vi "test-quintic-spline-02.vi"() -> (3 "Test Passed":bool)   [LabVIEW 2019]
uses:
  <vilib>/Rock Robotics/WPI/ThirdParty/JAS_Junk/TrajLib/POSEwCURVATURE.ctl
  <vilib>/Rock Robotics/WPI/ThirdParty/JAS_Junk/TrajLib/POSE2D.ctl
  <vilib>/Rock Robotics/WPI/ThirdParty/JAS_Junk/TrajLib/TRANSLATION2D.ctl
  <vilib>/Rock Robotics/WPI/ThirdParty/JAS_Junk/TrajLib/ROTATION2D.ctl
  <vilib>/Rock Robotics/WPI/ThirdParty/JAS_Junk/TrajLib/Rotation2d_CreateAngle.vi
  <vilib>/Rock Robotics/WPI/ThirdParty/JAS_Junk/TrajLib/Translation2d_Create.vi
  <vilib>/Rock Robotics/WPI/ThirdParty/JAS_Junk/TrajLib/Util_CalcDist.vi
  <vilib>/Rock Robotics/WPI/ThirdParty/JAS_Junk/TrajLib/Trajectory_Library.lvlib
panel:
  out "XY Graph":cluster{dbl[], dbl[]}(graph)
  out "Numb\nWaypoints":i32
  out "All Interior \nwayPoints\nFound (True)":bool
  out "end rot = 0":dbl
  out "end y = 0":dbl
  out "end x = 0":dbl
  out "start rot = 0":dbl
  out "start y = 0":dbl
  out "start x = 0":dbl
  out "max dtheta < 0.0872":dbl
  out "max dy < 0.00127":dbl
  out "max dx  < 0.127":dbl
  out "Overall Error":errorcluster
  out "Elements":i32
  out "Create Spline Error":errorcluster
  out "SplinePoses\nWCurve":T1[](array[typedef]) {"POSE"."ROTATION"."SIN" format="%13.4f"; "POSE"."ROTATION"."COS" format="%13.4f"; "POSE"."ROTATION"."VALUE" format="%13.4f"; "POSE"."TRANSLATION"."Y" format="%14.3f"; "POSE"."TRANSLATION"."X" format="%14.3f"}
  out "Elapsed Time":dbl
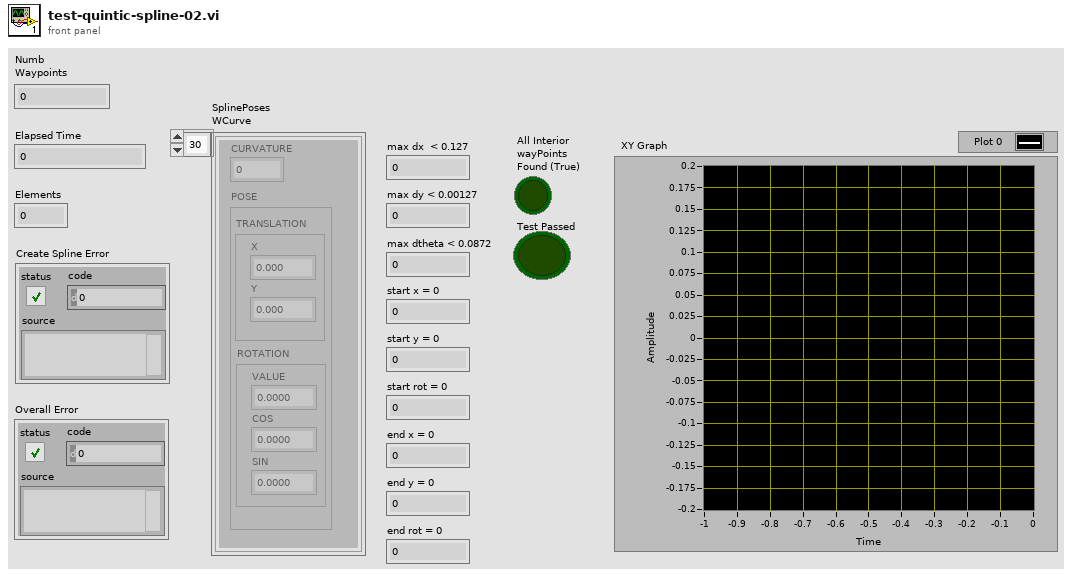
[diagram p1: front panel]
types:
  T1 = typedef "Trajectory_Library.lvlib/POSEwCURVATURE.ctl" = cluster{"CURVATURE":dbl, "POSE":T2}
  T2 = typedef "Trajectory_Library.lvlib/POSE2D.ctl" = cluster{"TRANSLATION":T3, "ROTATION":T4}
  T3 = typedef "Trajectory_Library.lvlib/TRANSLATION2D.ctl" = cluster{"X":dbl, "Y":dbl}
  T4 = typedef "Trajectory_Library.lvlib/ROTATION2D.ctl" = cluster{"VALUE":dbl, "COS":dbl, "SIN":dbl}
  T5 = typedef "Trajectory_Library.lvlib/SPLINE.ctl" = cluster{"Degree":i32, "Coefficients":T6}
  T6 = typedef "NI_Matrix.lvlib/RealMatrix.ctl" = dbl[][]
  T7 = typedef "Trajectory_Library.lvlib/TWIST2D.ctl" = cluster{"dX":dbl, "dY":dbl, "dTHETA":dbl}
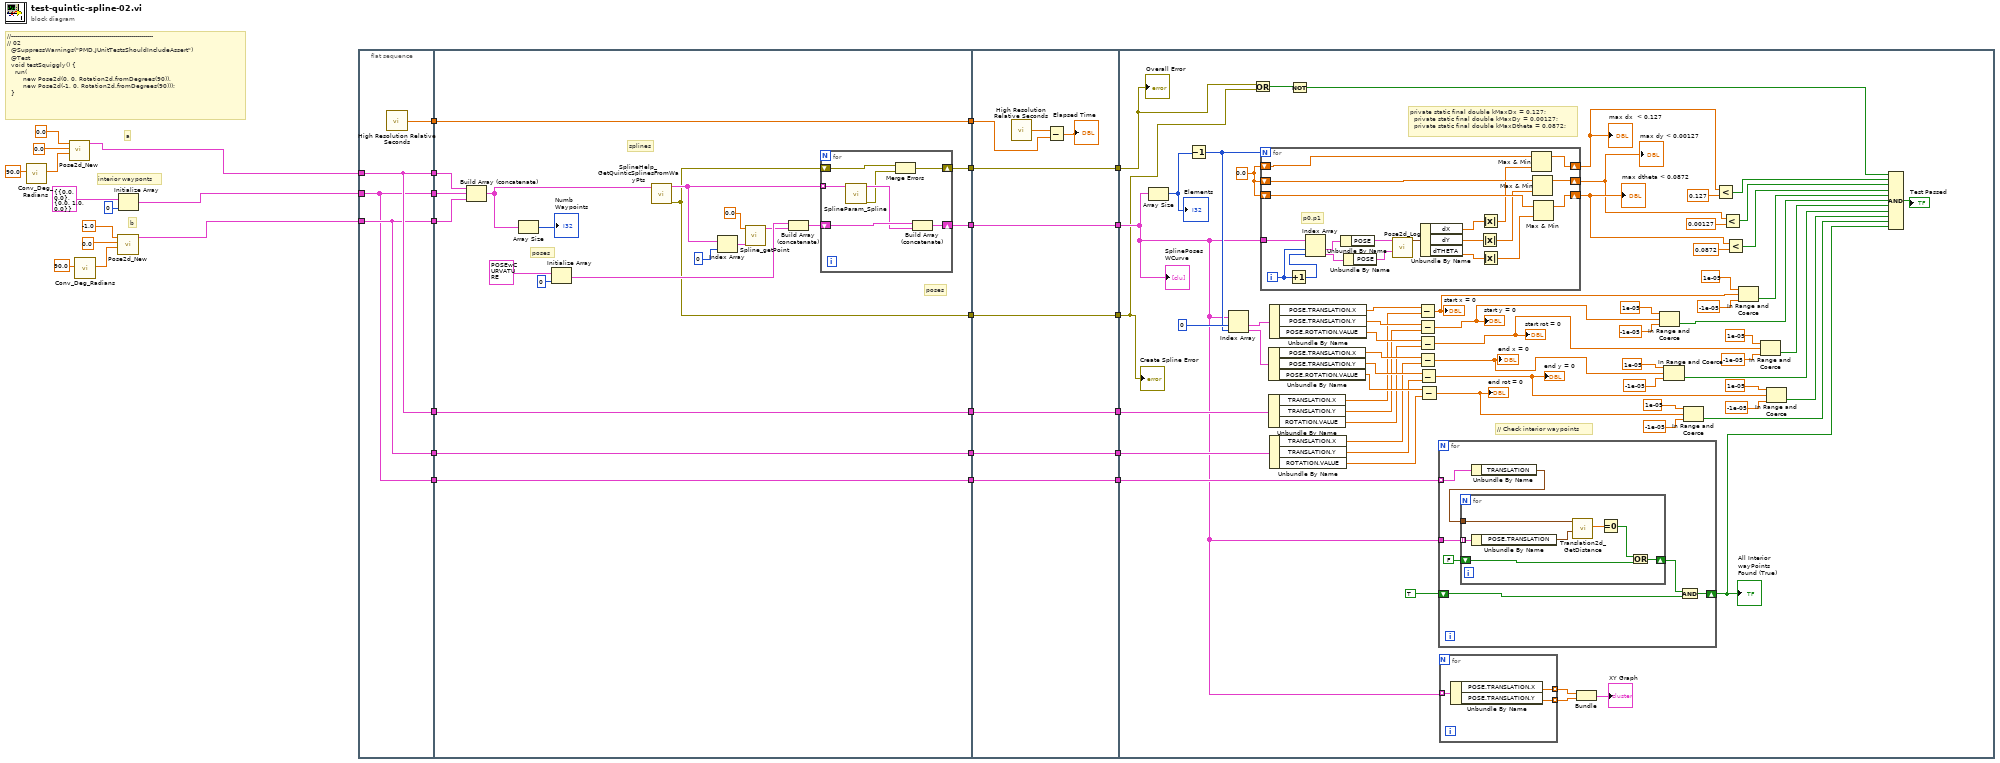
[diagram p0: block diagram]
diagram:
  # "interior wayponts"
  # "b"
  # "a"
  # "//-----------------------------------------------------------------------\n// 02\n  @SuppressWarnings(\"PMD.JUnitTestsShouldIncludeAssert\")\n  @Test\n  void testSquiggly() {\n    run(\n        new Pose2d(0, 0, Rotation2d.fromDegrees(90)),\n        new Pose2d(-1, 0, Rotation2d.fromDegrees(90)));\n  }"
  n1 = call <vilib>:"Conv_Deg_Radians.vi"("Degress"=90.0) -> ("Radians"=w6:dbl)  [unwired: 10 in]
  n2 = call <vilib>:"Pose2d_New.vi"("Heading"=w6, "Y"=0.0, "X"=0.0) -> ("out POSe"=w3:T2)  [unwired: 8 in]
  n3 = call <vilib>:"Conv_Deg_Radians.vi"("Degress"=90.0) -> ("Radians"=w9:dbl)  [unwired: 10 in]
  n4 = call <vilib>:"Pose2d_New.vi"("Heading"=w9, "Y"=0.0, "X"=-1.0) -> ("out POSe"=w1:T2)  [unwired: 8 in]
  n5 = Initialize Array(T2 {"TRANSLATION"={"X"=0.0, "Y"=0.0}, "ROTATION"={"VALUE"=0.0, "COS"=1.0, "SIN"=0.0}} ("POSE"), 0 ("dimension size")) -> (w2:T2[])
  n6 = flat-sequence {
    tunnel: w3 -> [w36]
    tunnel: [w36] -> w33
    tunnel: w1 -> [w35]
    tunnel: [w35] -> w32
    tunnel: [w37] -> w31
    tunnel: [w36] -> w23
    tunnel: [w35] -> w20
    tunnel: [w34] -> w15
    tunnel: w2 -> [w34]
    tunnel: [w34] -> w14
    tunnel: w33 -> [w42]
    tunnel: w32 -> [w41]
    tunnel: [w58] -> w30
    tunnel: w31 -> [w58]
    tunnel: [w48] -> w29
    tunnel: [w47] -> w27
    tunnel: [w46] -> w25
    tunnel: w23 -> [w45]
    tunnel: [w45] -> w22
    tunnel: w20 -> [w44]
    tunnel: [w44] -> w19
    tunnel: [w43] -> w16
    tunnel: w15 -> [w43]
    tunnel: w14 -> [w39]
    tunnel: w30 -> [w74]
    tunnel: w29 -> [w73]
    tunnel: [w73] -> w28
    tunnel: w27 -> [w72]
    tunnel: [w72] -> w26
    tunnel: w25 -> [w71]
    tunnel: [w71] -> w24
    tunnel: w22 -> [w68]
    tunnel: [w68] -> w21
    tunnel: w19 -> [w67]
    tunnel: [w67] -> w18
    tunnel: [w66] -> w17
    tunnel: w16 -> [w66]
    tunnel: w28 -> [w115]
    tunnel: w26 -> [w102]
    tunnel: w24 -> [w101]
    tunnel: w21 -> [w137]
    tunnel: w18 -> [w136]
    tunnel: w17 -> [w119]
    frame #0 {
      n7 = call <vilib>:"High Resolution Relative Seconds.vi"() -> ("relative seconds"=w37:dbl)
    }
    frame #1 {
      # "poses"
      # "poses"
      # "splines"
      n8 = Build Array (concatenate)(w42, w39, w41) -> (w38:T2[])
      n9 = Array Size(array=w38) -> (size(s)=→"Numb\nWaypoints":i32)
      n10 = Initialize Array(T1 {"CURVATURE"=0.0, "POSE"={"TRANSLATION"={"X"=0.0, "Y"=0.0}, "ROTATION"={"VALUE"=0.0, "COS"=1.0, "SIN"=0.0}}} ("POSEwCURVATURE"), 0 ("dimension size")) -> (w52:T1[])
      n11 = call <vilib>:"SplineHelp_GetQuinticSplinesFromWayPts.vi"("WayPoints"=w38) -> ("out Error"=w47:errorcluster, "Splines"=w49:T5[])  [unwired: 9 in]
      n12 = Index Array(array=w49, index=0) -> (element=w54:T5)
      n13 = call <vilib>:"Spline_getPoint.vi"("inputSPLINE"=w54, "Time"=0.0) -> ("POSEwCURVATURE"=w51:T1)  [unwired: 9 in]
      n14 = Build Array (concatenate)(w52, w51) -> (w50:T1[])
      n15 = for {
        shift-right: [w62] -> w48
        shift-left: w50 -> [w64]
        tunnel: w49 -> [w65] mode=indexing
        shift-right: [w60] -> w46
        shift-left: w47 -> [w61]
        n16 = call <vilib>:"SplineParam_Spline.vi"("inputSPLINE"=w65) -> ("error out"=w59:errorcluster, "outputPOSEwCURVATURE"=w63:T1[])  [unwired: 9 in]
        n17 = Merge Errors(w61, w59) -> (w60:errorcluster)
        n18 = Build Array (concatenate)(w64, w63) -> (w62:T1[])
      }
    }
    frame #2 {
      n19 = call <vilib>:"High Resolution Relative Seconds.vi"() -> ("relative seconds"=w69:dbl)
      n20 = Subtract(x=w69, y=w74) -> (x-y=→"Elapsed Time":dbl)
    }
    frame #3 {
      w138 = 0.0
      # "// Check interior waypoints"
      # "private static final double kMaxDx = 0.127;\n  private static final double kMaxDy = 0.00127;\n  private static final double kMaxDtheta = 0.0872;"
      n21 = Array Size(array=w115) -> (size(s)=w139:i32)
      "Elements" <- w139
      n22 = Decrement(x=w139) -> (x-1=w134:i32)
      n23 = Index Array(array=w115, index #1=0 ("index"), index #2=w134) -> (element #1=w133:T1, element #2=w132:T1)
      n24 = Or(x=w101, y=w102) -> (x .or. y?=w103:bool)
      n25 = for {
        N: w134 -> [_]
        tunnel: w115 -> [w174]
        shift-right: [w165] -> w107
        shift-left: w138 -> [w162]
        shift-right: [w163] -> w109
        shift-left: w138 -> [w160]
        shift-right: [w164] -> w108
        shift-left: w138 -> [w161]
        i -> [w176]
        # "p0,p1"
        n26 = Increment(x=w176) -> (x+1=w175:i32)
        n27 = Index Array(array=w174, index #1=w176, index #2=w175) -> (element #1=w173:T1, element #2=w172:T1)
        n28 = Unbundle By Name(w173) -> ("POSE"=w171:T2)
        n29 = Unbundle By Name(w172) -> ("POSE"=w170:T2)
        n30 = call <vilib>:"Pose2d_Log.vi"("end POSE"=w170, "in POSE"=w171) -> ("out TWIST"=w169:T7)  [unwired: 9 in]
        n31 = Unbundle By Name(w169) -> ("dX"=w166:dbl, "dY"=w167:dbl, "dTHETA"=w168:dbl)
        n32 = Absolute Value(x=w167) -> (abs(x)=w158:dbl)
        n33 = Absolute Value(x=w166) -> (abs(x)=w159:dbl)
        n34 = Absolute Value(x=w168) -> (abs(x)=w157:dbl)
        n35 = Max & Min(x=w162, y=w159) -> (max(x,y)=w165:dbl)  [unwired: 1 out]
        n36 = Max & Min(x=w161, y=w158) -> (max(x,y)=w164:dbl)  [unwired: 1 out]
        n37 = Max & Min(x=w160, y=w157) -> (max(x,y)=w163:dbl)  [unwired: 1 out]
      }
      "max dx  < 0.127" <- w107
      "max dy < 0.00127" <- w108
      "max dtheta < 0.0872" <- w109
      n38 = Unbundle By Name(w132) -> ("POSE.TRANSLATION.X"=w128:dbl, "POSE.TRANSLATION.Y"=w127:dbl, "POSE.ROTATION.VALUE"=w126:dbl)
      n39 = Unbundle By Name(w137) -> ("TRANSLATION.X"=w125:dbl, "TRANSLATION.Y"=w124:dbl, "ROTATION.VALUE"=w123:dbl)
      n40 = Unbundle By Name(w133) -> ("POSE.TRANSLATION.X"=w131:dbl, "POSE.TRANSLATION.Y"=w130:dbl, "POSE.ROTATION.VALUE"=w129:dbl)
      n41 = Unbundle By Name(w136) -> ("TRANSLATION.X"=w122:dbl, "TRANSLATION.Y"=w121:dbl, "ROTATION.VALUE"=w120:dbl)
      n42 = Not(x=w103) -> (.not. x?=w100:bool)
      n43 = Subtract(x=w131, y=w125) -> (x-y=w96:dbl)
      "start x = 0" <- w96
      n44 = Subtract(x=w130, y=w124) -> (x-y=w75:dbl)
      "start y = 0" <- w75
      n45 = Subtract(x=w129, y=w123) -> (x-y=w79:dbl)
      "start rot = 0" <- w79
      n46 = Subtract(x=w128, y=w122) -> (x-y=w80:dbl)
      "end x = 0" <- w80
      n47 = Subtract(x=w127, y=w121) -> (x-y=w87:dbl)
      "end y = 0" <- w87
      n48 = Subtract(x=w126, y=w120) -> (x-y=w91:dbl)
      "end rot = 0" <- w91
      n49 = for {
        tunnel: w119 -> [w144] mode=indexing
        tunnel: w115 -> [w149]
        shift-right: [w148] -> w99
        shift-left: TRUE -> [w147]
        n50 = Unbundle By Name(w144) -> ("TRANSLATION"=w143:T3)
        n51 = for {
          tunnel: w149 -> [w153] mode=indexing
          shift-right: [w156] -> w145
          shift-left: FALSE -> [w155]
          tunnel: w143 -> [w154]
          n52 = Unbundle By Name(w153) -> ("POSE.TRANSLATION"=w152:T3)
          n53 = call <vilib>:"Translation2d_GetDistance.vi"("other Translation"=w152, "In Translation"=w154) -> ("Distance"=w151:dbl)  [unwired: 9 in]
          n54 = Equal To 0?(x=w151) -> (x = 0?=w150:bool)
          n55 = Or(x=w150, y=w155) -> (x .or. y?=w156:bool)
        }
        n56 = And(x=w145, y=w147) -> (x .and. y?=w148:bool)
      }
      "All Interior \nwayPoints\nFound (True)" <- w99
      n57 = for {
        tunnel: [w142] -> w117 mode=indexing
        tunnel: [w141] -> w116 mode=indexing
        tunnel: w115 -> [w140] mode=indexing
        n58 = Unbundle By Name(w140) -> ("POSE.TRANSLATION.X"=w142:dbl, "POSE.TRANSLATION.Y"=w141:dbl)
      }
      n59 = Bundle(w117, w116) -> (→"XY Graph":cluster{dbl[], dbl[]})  [unwired: 1 in]
      n60 = In Range and Coerce(upper limit=1e-05, x=w75, lower limit=-1e-05) -> (In Range?=w76:bool)  [unwired: 1 out]
      n61 = In Range and Coerce(upper limit=1e-05, x=w80, lower limit=-1e-05) -> (In Range?=w82:bool)  [unwired: 1 out]
      n62 = In Range and Coerce(upper limit=1e-05, x=w91, lower limit=-1e-05) -> (In Range?=w92:bool)  [unwired: 1 out]
      n63 = Less?(x=w107, y=0.127) -> (x < y?=w106:bool)
      n64 = Less?(x=w108, y=0.00127) -> (x < y?=w105:bool)
      n65 = Less?(x=w109, y=0.0872) -> (x < y?=w104:bool)
      n66 = In Range and Coerce(upper limit=1e-05, x=w96, lower limit=-1e-05) -> (In Range?=w95:bool)  [unwired: 1 out]
      n67 = In Range and Coerce(upper limit=1e-05, x=w79, lower limit=-1e-05) -> (In Range?=w81:bool)  [unwired: 1 out]
      n68 = In Range and Coerce(upper limit=1e-05, x=w87, lower limit=-1e-05) -> (In Range?=w88:bool)  [unwired: 1 out]
      n69 = Compound Arithmetic op=AND(w100, w106, w105, w104, w95, w76, w81, w82, w88, w92, w99) -> (→"Test Passed":bool)
      "SplinePoses\nWCurve" <- w115
      "Create Spline Error" <- w102
      "Overall Error" <- w101
    }
  }
